vi "triggering.vi"() -> ()   [LabVIEW 2021]
uses:
  <vilib>/DAQmx/read.llb/DAQmx Read (Analog Wfm 1Chan NSamp).vi
  <vilib>/DAQmx/create/channels.llb/DAQmx Create Channel (AI-Voltage-Basic).vi
  <vilib>/DAQmx/configure/timing.llb/DAQmx Timing (Sample Clock).vi
  <vilib>/DAQmx/configure/trigger.llb/DAQmx Reference Trigger (Digital Edge).vi
  <vilib>/DAQmx/miscellaneous.llb/DAQmx Fill In Error Info.vi
panel:
  in  "rate":dbl=1000.0 format="%0.2f"
  in  "pretrigger samples per channel":u32=500
  out "Waveform Graph":waveform(dbl)(graph)
  in  "# samples to read":i32=1000
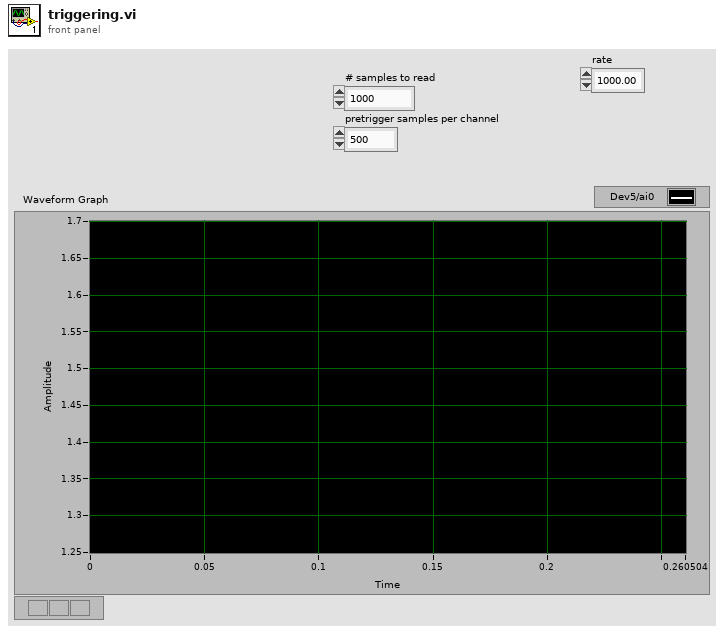
[diagram p1: front panel]
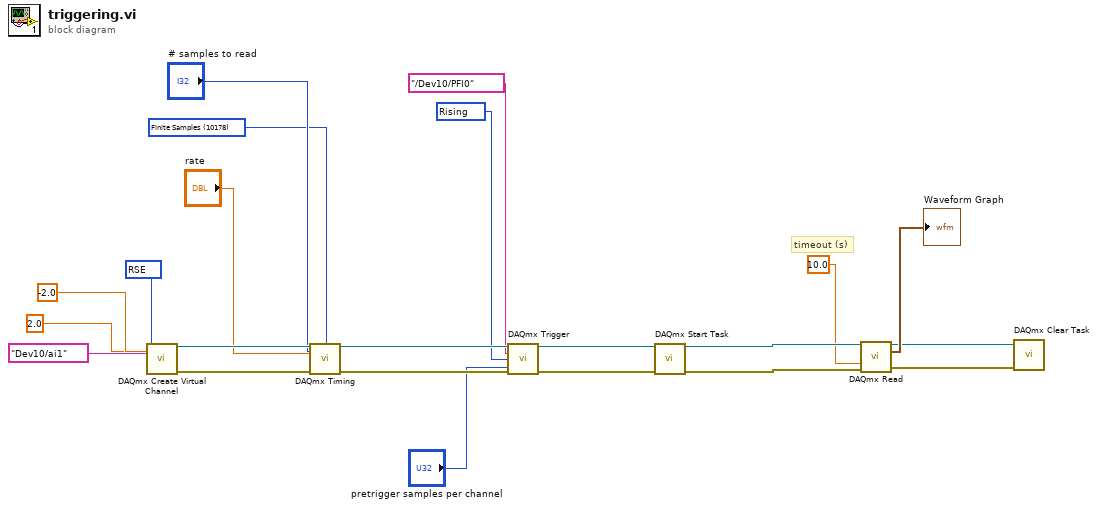
[diagram p0: block diagram]
diagram:
  w13 = 10083 items=["Default"=-1, "RSE"=10083, "NRSE"=10078, "Differential"=10106, "Pseudodifferential"=12529] ("input terminal configuration")
  w14 = 10178 items=["Finite Samples"=10178, "Continuous Samples"=10123, "Hardware Timed Single Point"=12522] ("sample mode")
  w15 = 10280 items=["Rising"=10280, "Falling"=10171] ("edge")
  # "timeout (s)"
  n1 = call-poly <vilib>:"DAQmx Create Virtual Channel.vi"("maximum value"=2.0, "minimum value"=-2.0, "input terminal configuration"=w13, "physical channels"=tag "Dev10/ai1") -> ("task out"=w19:refnum<k21>, "error out"=w22:errorcluster)  [unwired: 10 in]
  n2 = call-poly <vilib>:"DAQmx Timing.vi"("task/channels in"=w19, "sample mode"=w14, "samples per channel"="# samples to read", "rate"="rate", "error in"=w22) -> ("task out"=w18:refnum<k21>, "error out"=w21:errorcluster)  [unwired: 9 in]
  n3 = call-poly <vilib>:"DAQmx Trigger.vi"("task/channels in"=w18, "source"=tag "/Dev10/PFI0", "edge"=w15, "error in"=w21, "pretrigger samples per channel"="pretrigger samples per channel") -> ("task out"=w17:refnum<k21>, "error out"=w20:errorcluster)  [unwired: 9 in]
  n4 = call <vilib>:"DAQmx Start Task.vi"("task/channels in"=w17, "error in"=w20) -> ("task out"=w7:refnum<k21>, "error out"=w8:errorcluster)  [unwired: 12 in]
  n5 = call-poly <vilib>:"DAQmx Read.vi"("task/channels in"=w7, "timeout"=10.0, "error in"=w8) -> ("task out"=w4:refnum<k21>, "data"=→"Waveform Graph":waveform(dbl), "error out"=w3:errorcluster)  [unwired: 10 in]
  n6 = call <vilib>:"DAQmx Clear Task.vi"("task in"=w4, "error in"=w3) -> ()  [unwired: 13 in, 1 out]
